vi "Kpro Read String Pot 2016.vi"(0 "Read String Pot":bool, 1 "Feet of\nStainless to be\nUsed (Count) in":i32, 2 "Session Array in":dbl[][](array[numeric]), 3 "Flow":dbl, 4 "Manual Depth In":dbl, 5 "Finished In":bool, 6 "Depth Cluster in":T1, 7 "error in (no error)":errorcluster, 8 "String Pot \nSlope in":dbl=1.7339999675750732 format="%.2f", 9 "Sensor Cluster In in":T2, 10 "Descriptions":string[](array[string]), 11 "Pressure in":dbl format="%.2f", 12 "Array in":refnum<k24>[](array[refnum]), 13 "Downhole Pressure Sensor":dbl format="%#_13g", 14 "Initial Measurement Input":bool, 15 "Downhole Pressure (V)":dbl, 16 "Aux3 Slope In":dbl) -> (17 "DHT IK Out":dbl, 18 "Sensor Cluster 2":T2, 19 "IK":dbl, 20 "Array out":refnum<k24>[](array[refnum]), 21 "Generate Array Calc IK":bool, 22 "Filter Output":dbl, 23 "Depth Cluster  2":T1, 24 "Feet of\nStainless to be\nUsed (Count) out":i32, 25 "Depth Cluster out":T1, 26 "Single String Pot Session Array out":dbl[][](array[numeric]), 27 "error out":errorcluster)   [LabVIEW 2016]
uses:
  controls/MCC DAQ Readings.ctl
  C:/Cascade-lv16-64/builds/Waterloo Main Program/cascade/data/ULx_LV.dll
  builds/Waterloo Main Program/cascade/data/ULx_LV.dll
  controls/Kpro hydraulic measurement cluster.ctl
panel:
  out "finished take data update depth":bool
  out "Aux3\\EC Out":dbl
  in  "DHT IK In":dbl
  out "Manual measurement triggered":bool
  out "Depth Rate":dbl format="%.2f"
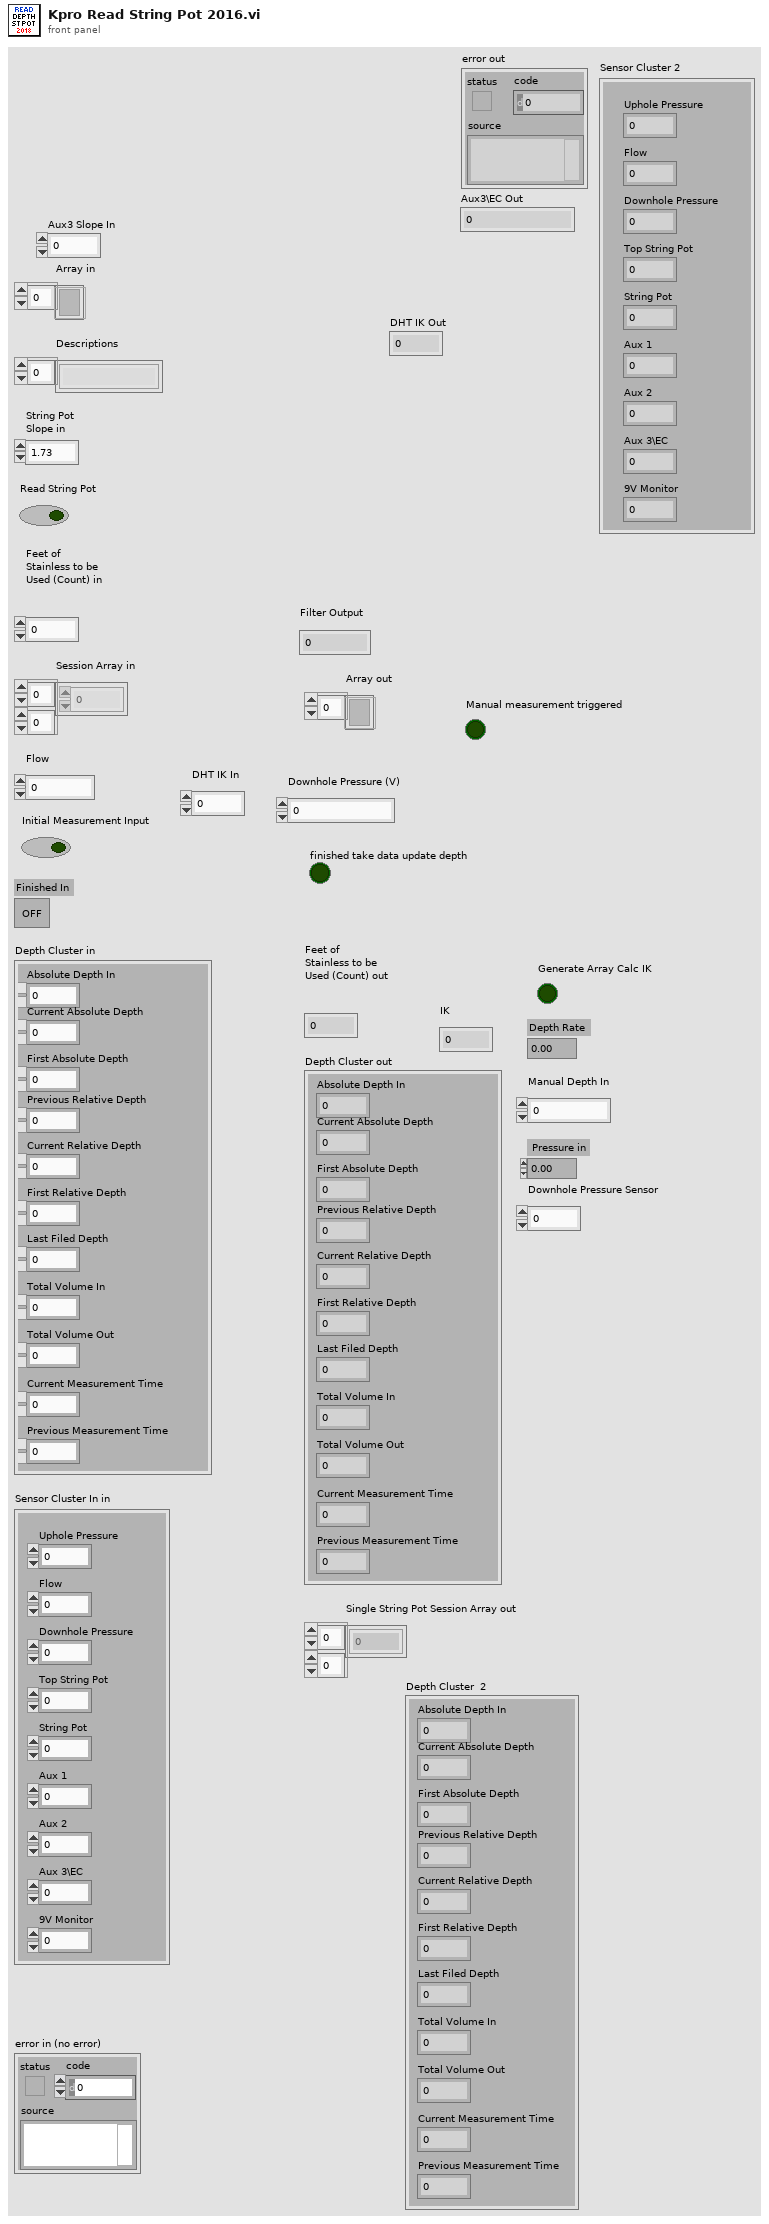
[diagram p1: front panel]
types:
  T1 = typedef "Kpro hydraulic measurement cluster.ctl" = cluster{"Absolute Depth In":dbl, "Current Absolute Depth":dbl, "First Absolute Depth":dbl, "Previous Relative Depth":dbl, "Current Relative Depth":dbl, "First Relative Depth":dbl, "Last Filed Depth":dbl, "Total Volume In":dbl, "Total Volume Out":dbl, "Current Measurement Time":dbl, "Previous Measurement Time":dbl}
  T2 = typedef "MCC DAQ Readings.ctl" = cluster{"Uphole Pressure":dbl, "Flow":dbl, "Downhole Pressure":dbl, "Top String Pot":dbl, "String Pot":dbl, "Aux 1":dbl, "Aux 2":dbl, "Aux 3\\EC":dbl, "9V Monitor":dbl}
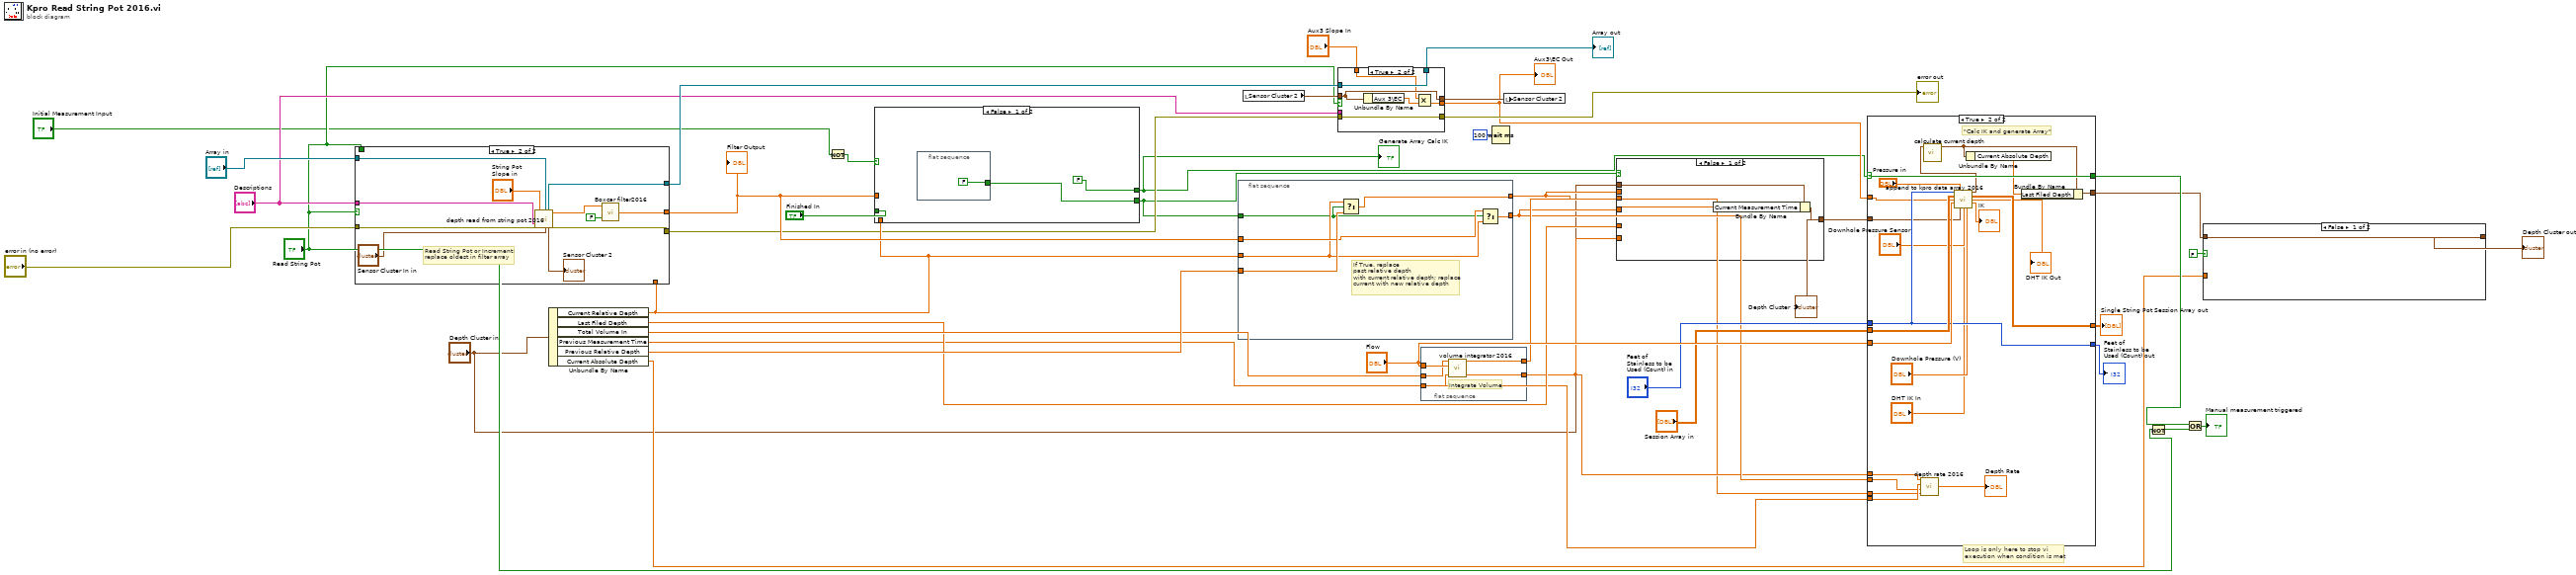
[diagram p0: block diagram]
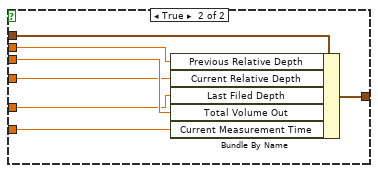
[diagram p2: hidden frame]
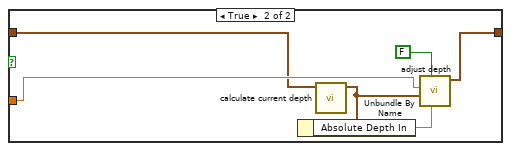
[diagram p3: hidden frame]
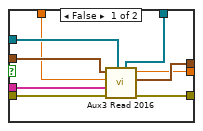
[diagram p4: hidden frame]
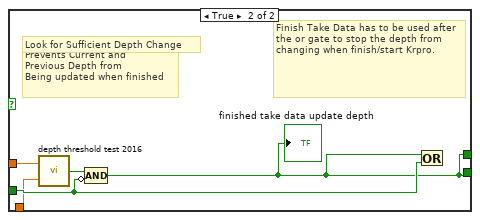
[diagram p5: hidden frame]
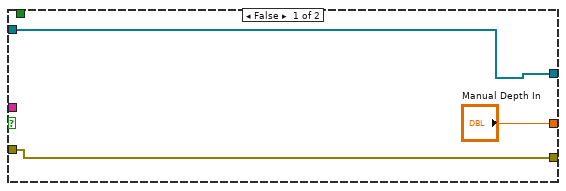
[diagram p6: hidden frame]
diagram:
  # "Loop is only here to stop vi \nexecution when condition is met"
  n1 = Unbundle By Name("Depth Cluster in") -> ("Current Relative Depth"=w30:dbl, "Last Filed Depth"=w31:dbl, "Total Volume In"=w34:dbl, "Previous Measurement Time"=w23:dbl, "Previous Relative Depth"=w36:dbl, "Current Absolute Depth"=w8:dbl)
  n2 = case shown="True" "Read String Pot" {
    tunnel: ["Manual Depth In" w55] -> w33
    tunnel: "Read String Pot" -> [_ _]
    tunnel: "Descriptions" -> [_ w54]
    tunnel: [w45 w52] -> w20
    tunnel: "Array in" -> [w45 w51]
    tunnel: w30 -> [_ _]
    tunnel: "error in (no error)" -> [w43 w47]
    tunnel: [w43 w46] -> w17
    frame False {
    }
    frame True {
      # "Read String Pot or Increment;\nreplace oldest in filter array"
      n3 = call "depth read from string pot 2016.vi"("Descriptions"=w54, "error in (no error)"=w47, "String Pot \nSlope"="String Pot \nSlope in", "Array in"=w51, "Sensor Cluster In"="Sensor Cluster In in") -> ("Array out"=w52:refnum<k24>[], "Sensor Cluster 2"=→"Sensor Cluster 2":T2, "Depth"=w56:dbl, "error out"=w46:errorcluster)  [unwired: 11 in]
      n4 = call "Boxcar filter2016.vi"("Initialize"=FALSE, "Filter Input"=w56) -> ("Filter Output"=w55:dbl)  [unwired: 1 in]
    }
  }
  "Filter Output" <- w33
  n5 = Not(x="Initial Measurement Input") -> (.not. x?=w25:bool)
  n6 = case shown="False" w25 {
    tunnel: [w58 w60] -> w1
    tunnel: "Finished In" -> [_ w63]
    tunnel: w33 -> [_ w62]
    tunnel: w30 -> [_ w61]
    tunnel: [FALSE w60] -> w9
    frame False {
      n7 = flat-sequence {
        tunnel: [FALSE] -> w58
        frame #0 {
        }
      }
    }
    frame True {
      # "Finish Take Data has to be used after the or gate to stop the depth from changing when finish/start Krpro."
      # "Look for Sufficient Depth Change"
      # "This Funky Gate\nPrevents Current and \nPrevious Depth from \nBeing updated when finished"
      n8 = call "depth threshold test 2016.vi"("Depth\nPrevious"=w61, "Depth \nCurrent"=w62) -> ("Threshold\nExceeded"=w64:bool)
      n9 = Compound Arithmetic op=AND(w64, invert w63) -> (w60:bool)
      "finished take data update depth" <- w60
      n10 = Or(x=w60, y=w63) -> ()  [unwired: 1 out]
    }
  }
  "Generate Array Calc IK" <- w9
  n11 = flat-sequence {
    tunnel: [w70] -> w21
    tunnel: w36 -> [w69]
    tunnel: [w68] -> w24
    tunnel: w1 -> [w65]
    tunnel: w33 -> [w67]
    tunnel: w30 -> [w66]
    frame #0 {
      # "If True, replace\npast relative depth\nwith current relative depth; replace\ncurrent with new relative depth"
      n12 = Select(t=w66, s=w65, f=w69) -> (s? t:f=w70:dbl)
      n13 = Select(t=w67, s=w65, f=w66) -> (s? t:f=w68:dbl)
    }
  }
  n14 = local read "Sensor Cluster 2"() -> (w14:T2)
  n15 = case shown="True" "Read String Pot" {
    tunnel: w20 -> [w79 w84]
    tunnel: [w78 w84] -> w19
    tunnel: w17 -> [w77 w85]
    tunnel: [w76 w85] -> w16
    tunnel: [w75 w83] -> w15
    tunnel: w14 -> [w74 w83]
    tunnel: "Descriptions" -> [w73 _]
    tunnel: "Aux3 Slope In" -> [w72 w80]
    tunnel: [w71 w81] -> w11
    frame False {
      n16 = call "Aux3 Read 2016.vi"("Array in"=w79, "error in (no error)"=w77, "Descriptions"=w73, "Aux3 Slope In"=w72, "Sensor Cluster"=w74) -> ("error out"=w76:errorcluster, "Sensor Cluster 2"=w75:T2, "Aux3\\EC Out"=w71:dbl, "Array out"=w78:refnum<k24>[])  [unwired: 3 in]
    }
    frame True {
      n17 = Unbundle By Name(w83) -> ("Aux 3\\EC"=w82:dbl)
      n18 = Multiply(x=w80, y=w82) -> (x*y=w81:dbl)
    }
  }
  "Array out" <- w19
  "error out" <- w16
  "Aux3\\EC Out" <- w11
  n19 = flat-sequence {
    tunnel: w23 -> [w90]
    tunnel: [w89] -> w22
    tunnel: "Flow" -> [w88]
    tunnel: w34 -> [w87]
    tunnel: [w86] -> w35
    frame #0 {
      # "Integrate Volume"
      n20 = call "volume integrator 2016.vi"("Previous Time (sec)"=w90, "Flow"=w88, "Total Volume in"=w87) -> ("Current Time (sec)"=w89:dbl, "Total Volume Out mL"=w86:dbl)  [unwired: 3 in]
    }
  }
  n21 = Wait (ms)(milliseconds to wait=u32 100) -> ()  [unwired: 1 out]
  n22 = local write "Sensor Cluster 2"(w15) -> ()
  n23 = case shown="False" w1 {
    tunnel: w35 -> [_ w100]
    tunnel: w31 -> [_ w99]
    tunnel: w24 -> [_ w98]
    tunnel: w22 -> [w91 w97]
    tunnel: w21 -> [_ w96]
    tunnel: [w92 w95] -> w7
    tunnel: "Depth Cluster in" -> [w93 w94]
    frame False {
      n24 = Bundle By Name(cluster=w93, "Current Measurement Time"=w91) -> (w92:T1)
    }
    frame True {
      n25 = Bundle By Name(cluster=w94, "Previous Relative Depth"=w96, "Current Relative Depth"=w98, "Last Filed Depth"=w99, "Total Volume Out"=w100, "Current Measurement Time"=w97) -> (w95:T1)
    }
  }
  "Depth Cluster  2" <- w7
  n26 = case shown="True" w9 {
    selector: w9 -> [w102 w120]
    tunnel: "Session Array in" -> [w101 w126]
    tunnel: [w101 w125] -> w38
    tunnel: "Feet of\nStainless to be\nUsed (Count) in" -> [w103 w122]
    tunnel: "Flow" -> [_ w124]
    tunnel: [w104 w119] -> w6
    tunnel: w7 -> [w104 w118]
    tunnel: [w103 w122] -> w41
    tunnel: [w102 w120] -> w29
    tunnel: w24 -> [_ w110]
    tunnel: w23 -> [_ w111]
    tunnel: w22 -> [_ w109]
    tunnel: w21 -> [_ w108]
    tunnel: w11 -> [_ w107]
    frame False {
    }
    frame True {
      # "\"Calc IK and generate Array\""
      n27 = call "depth rate 2016.vi"("Depth Last"=w108, "Depth Current"=w110, "Time Last"=w111, "Time Current"=w109) -> ("Depth Rate"=→"Depth Rate":dbl)
      n28 = call "append to kpro data array 2016.vi"("Feet of\nStainless to be\nUsed (Count) in"=w122, "Up hole Pressure Sensor"="Pressure in", "DHT IK"="DHT IK In", "Corrected Array in"=w126, "Aux3/EC"=w107, "Flow"=w124, "Cluster in"=w118, "Downhole Pressure Sensor"="Downhole Pressure Sensor", "Downhole Pressure (V)"="Downhole Pressure (V)") -> ("Cluster out 2"=w117:T1, "Array Out"=w125:dbl[][], "DHT IK Out"=→"DHT IK Out":dbl, "IK"=→"IK":dbl)  [unwired: 2 in, 1 out]
      n29 = call "calculate current depth.vi"("Cluster in"=w117) -> ("Cluster out"=w116:T1)  [unwired: 10 in]
      n30 = Unbundle By Name(w116) -> ("Current Absolute Depth"=w115:dbl)
      n31 = Bundle By Name(cluster=w116, "Last Filed Depth"=w115) -> (w119:T1)
    }
  }
  "Feet of\nStainless to be\nUsed (Count) out" <- w41
  "Single String Pot Session Array out" <- w38
  n32 = Not(x="Read String Pot") -> (.not. x?=w26:bool)
  n33 = Or(x=w29, y=w26) -> (x .or. y?=→"Manual measurement triggered":bool)
  n34 = case shown="False" FALSE {
    tunnel: w6 -> [w127 w128]
    tunnel: [w127 w129] -> w5
    tunnel: w8 -> [_ w131]
    frame False {
    }
    frame True {
      n35 = call "calculate current depth.vi"("Cluster in"=w128) -> ("Cluster out"=w133:T1)  [unwired: 10 in]
      n36 = Unbundle By Name(w133) -> ("Absolute Depth In"=w132:dbl)
      n37 = call "adjust depth.vi"("Current Depth"=w132, "Read String Pot"=FALSE, "Depth Cluster"=w133, "Depth to \nbe Used \n(Feet)"=w131) -> ("Cluster out"=w129:T1)  [unwired: 7 in]
    }
  }
  "Depth Cluster out" <- w5
